vi "Set Object Entry.vi"(8 "error in":errorcluster, 9 "Obj Entry":refnum<class "Object Entry.lvclass">, 11 "Obj Dict in":refnum<class "Object Dictionary.lvclass">) -> (0 "error out":errorcluster, 3 "Obj Dict out":refnum<class "Object Dictionary.lvclass">)   [LabVIEW 2020, in "CANopen.lvlib" / "Object Dictionary.lvclass"]
uses:
  Object Dictionary.lvclass
  Object Dictionary.lvclass/Object Dictionary.ctl
  Object Entry/Object Entry.lvclass
  Ordered-Dictionary/Ordered Object Dictionary/Source/Ordered Object Dictionary.lvclass
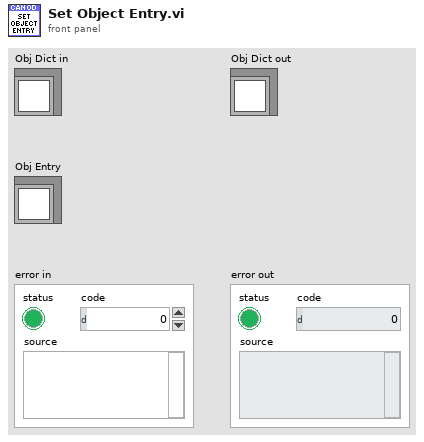
[diagram p1: front panel]
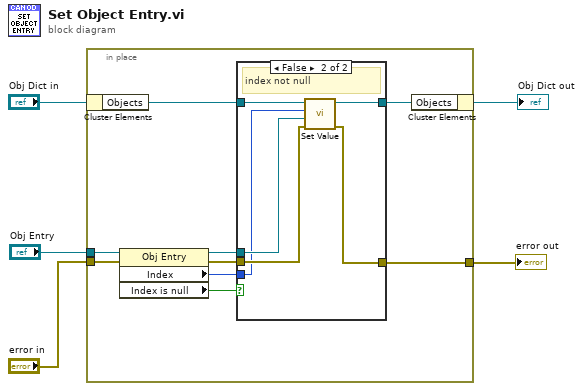
[diagram p0: block diagram]
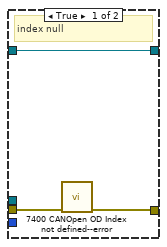
[diagram p2: hidden frame]
diagram:
  n1 = in-place {
    in-place-border: "error in" -> [w9]
    in-place-border: [w13] -> w2
    in-place-border: "Obj Entry" -> [w11]
    n2 = in-place-cluster #1("Obj Dict in") -> ("Objects"=w14:refnum<class "Ordered Object Dictionary.lvclass">)
    n3 = property class="Obj Entry"(reference=w11, error in=w9) -> (reference out=w10:refnum<class "Object Entry.lvclass">, error out=w8:errorcluster, "Index"=w6:u16, "Index is null"=w7:bool)
    n4 = case shown="False" w7 {
      tunnel: w14 -> [w16 w23]
      tunnel: [w15 w22] -> w13
      tunnel: [w16 w21] -> w12
      tunnel: w10 -> [_ w20]
      tunnel: w8 -> [w17 w19]
      tunnel: w6 -> [_ w18]
      frame True {
        # "index null"
        n5 = call "7400 CANOpen OD Index not defined--error.vi"("error in"=w17) -> ("error out"=w15:errorcluster)  [unwired: 9 in, 1 out]
      }
      frame False {
        # "index not null"
        n6 = call "Set Value.vi"("error in"=w19, "Value"=w20, "Key"=w18, "Ordered Object Dictionary in"=w23) -> ("error out"=w22:errorcluster, "Ordered Object Dictionary out"=w21:refnum<class "Ordered Object Dictionary.lvclass">)  [unwired: 6 in]
      }
    }
    n7 = in-place-cluster #1("Objects"=w12) -> (→"Obj Dict out":refnum<class "Object Dictionary.lvclass">)
  }
  "error out" <- w2
